vi "test Parse EST Clusters into EST IP.vi"(8 "error in (no error)":errorcluster, 11 "TestCase in":refnum<class "Bitfile Parsing Test Case.lvclass">) -> (0 "error out":errorcluster, 3 "TestCase out":refnum<class "Bitfile Parsing Test Case.lvclass">)   [LabVIEW 2015, in "Bitfile Parsing Test Case.lvclass"]
uses:
  Bitfile Parsing Test Case.lvclass
  <userlib>/_OpenG.lib/file/file.llb/Append Path to Root if Relative - Scalar__ogtk.vi
  <vilib>/addons/_JKI Toolkits/VI Tester/TestCase.llb/TestCase.lvclass
  System Explorer/Engine Simulation Toolkit System Explorer.lvlib
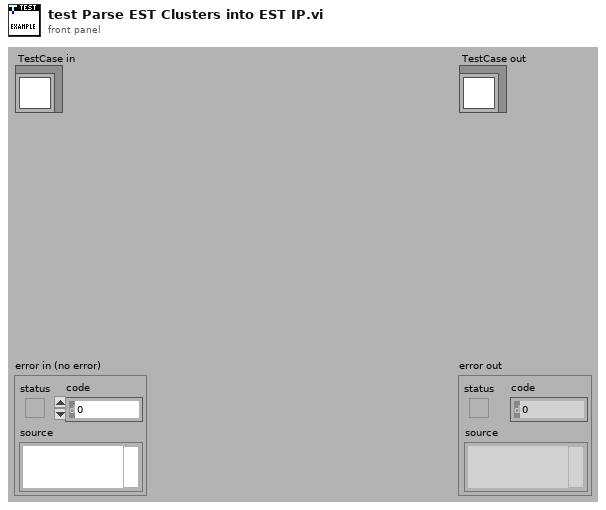
[diagram p1: front panel]
types:
  T1 = typedef "Engine Simulation Toolkit Shared.lvlib/Bitfile EST Version.ctl" = enum16{"1.0", "1.1", "1.2", "1.3"}
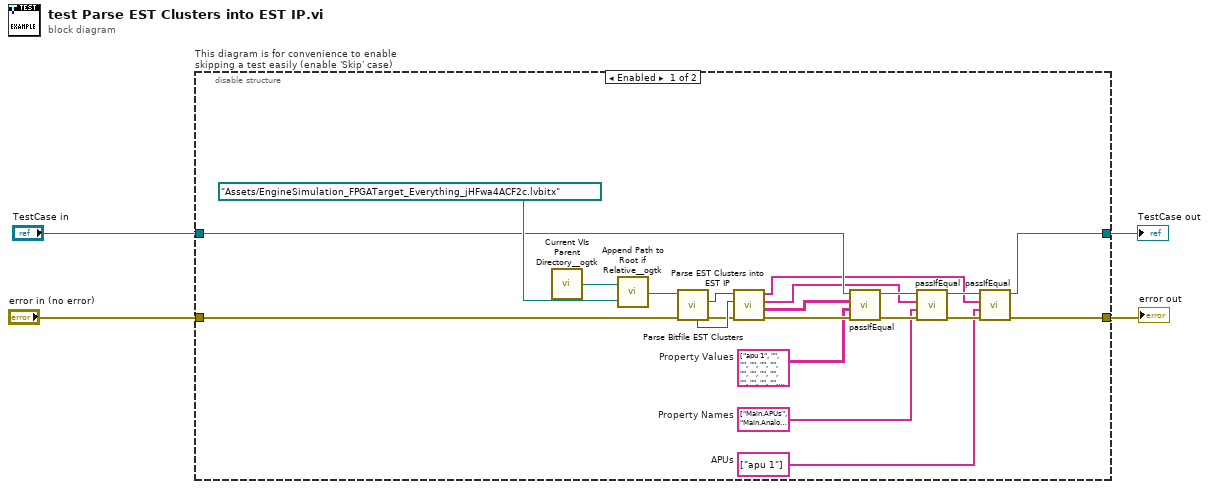
[diagram p0: block diagram]
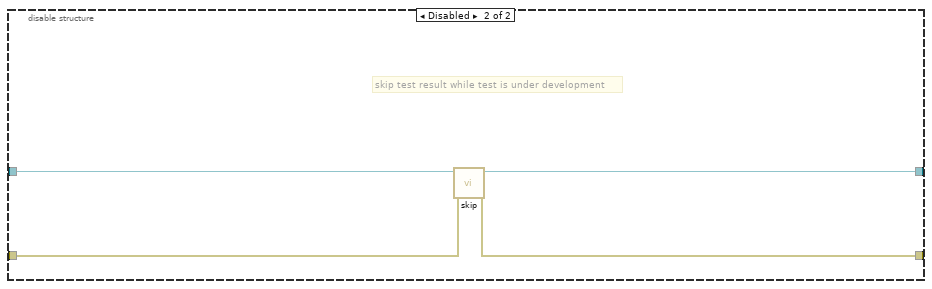
[diagram p2: hidden frame]
diagram:
  n1 = disable-structure "This diagram is for convenience to enable skipping a test easily (enable 'Skip' case)" shown="Enabled" {
    disable-tunnel: "TestCase in" -> [w17 w29]
    disable-tunnel: [w7 w27] -> w1
    disable-tunnel: [w9 w28] -> w3
    disable-tunnel: "error in (no error)" -> [w22 w26]
    frame Enabled {
      w16 = string[][] [["apu 1", "", "", "", "", "", "", "", "", "", "", "", "", "", "", "", "", "", "", "", "", "", "", "", "", "", "", "", "", ""], ["replay AO 0", "replay AO 1", "", "", "", "", "", "", "", "", "", "", "", "", "", "", "", "", "", "", "", "", "", "", "", "", "", "", "", ""], ["Pattern DIO 0", "Pattern DIO 1", "Pattern DIO 2", "Pattern DIO 3", "", "", "", "", "", "", "", "", "", "", "", "", "", "", "", "", "", "", "", "", "", "", "", "", "", ""], ["Event DIO 4.Event 1", "Event DIO 5.Event 1", "Event DIO 6.Event 1", "Event DIO 7.Event 1", "Event DIO 8.Event 1", "Event DIO 9.Event 1", "Multi Event DIO 10.Event 1", "Multi Event DIO 10.Event 2", "Multi Event DIO 10.Event 3", "Multi Event DIO 10.Event 4", "Multi Event DIO 11.Event 1", "Multi Event DIO 11.Event 2", "Multi Event DIO 11.Event 3", "Multi Event DIO 11.Event 4", "Multi Event DIO 12.Event 1", "Multi Event DIO 12.Event 2", "Multi Event DIO 12.Event 3", "Multi Event DIO 12.Event 4", "Multi Event DIO 13.Event 1", "Multi Event DIO 13.Event 2", "Multi Event DIO 13.Event 3", "Multi Event DIO 13.Event 4", "Multi Event DIO 14.Event 1", "Multi Event DIO 14.Event 2", "Multi Event DIO 14.Event 3", "Multi Event DIO 14.Event 4", "Multi Event DIO 15.Event 1", "Multi Event DIO 15.Event 2", "Multi Event DIO 15.Event 3", "Multi Event DIO 15.Event 4"], ["Event DIO 4", "Event DIO 5", "Event DIO 6", "Event DIO 7", "Event DIO 8", "Event DIO 9", "Multi Event DIO 10", "Multi Event DIO 11", "Multi Event DIO 12", "Multi Event DIO 13", "Multi Event DIO 14", "Multi Event DIO 15", "", "", "", "", "", "", "", "", "", "", "", "", "", "", "", "", "", ""], ["Knock AO 2.Cylinder 1", "Knock AO 2.Cylinder 2", "Knock AO 2.Cylinder 3", "Knock AO 2.Cylinder 4", "Knock AO 2.Cylinder 5", "Knock AO 2.Cylinder 6", "Knock AO 3.Cylinder 1", "Knock AO 3.Cylinder 2", "Knock AO 3.Cylinder 3", "Knock AO 3.Cylinder 4", "Knock AO 3.Cylinder 5", "Knock AO 3.Cylinder 6", "", "", "", "", "", "", "", "", "", "", "", "", "", "", "", "", "", ""], ["Knock AO 2", "Knock AO 3", "", "", "", "", "", "", "", "", "", "", "", "", "", "", "", "", "", "", "", "", "", "", "", "", "", "", "", ""], ["Dir Speed DIO0", "Dir Speed DIO1", "", "", "", "", "", "", "", "", "", "", "", "", "", "", "", "", "", "", "", "", "", "", "", "", "", "", "", ""]]  # Property Values
      w11 = string[] ["Main.APUs", "Main.Analog Replays", "Main.Digital PatGens", "Main.ETiming Caps", "Main.ETiming Meas", "Main.Knock Cylinder", "Main.Knock Sensor", "Main.DirSpeed Sensor"]  # Property Names
      w5 = string[] ["apu 1"]  # APUs
      n2 = call <userlib>:"Current VIs Parent Directory__ogtk.vi"() -> ("Parent Directory (+ Relative)"=w25:path)  [unwired: 5 in]
      n3 = call-poly <userlib>:"Append Path to Root if Relative__ogtk.vi"("Absolute or Relative Path"=path "Assets/EngineSimulation_FPGATarget_Everything_jHFwa4ACF2c.lvbitx" ("bitfile path"), "Root Path"=w25) -> ("Absolute or Appended Path"=w23:path)
      n4 = call "Parse Bitfile EST Clusters.vi"("error in (no error)"=w22, "bitfile path"=w23) -> ("error out"=w19:errorcluster, "EPS IP LUT"=w21:variant, "EST version enum"=w20:T1)  [unwired: 5 in, 2 out]
      n5 = call "Parse EST Clusters into EST IP.vi"("error in (no error)"=w19, "EST version enum"=w20, "EPS IP LUT"=w21) -> ("error out"=w18:errorcluster, "Property Values"=w15:string[][], "Property Names"=w12:string[], "APUs"=w6:string[])  [unwired: 5 in]
      n6 = call-dynamic "passIfEqual.vi"("error in (no error)"=w18, "y"=w16, "x"=w15, "TestCase in"=w17) -> ("error out"=w14:errorcluster, "TestCase out"=w13:refnum<class "Bitfile Parsing Test Case.lvclass">)  [unwired: 6 in]
      n7 = call-dynamic "passIfEqual.vi"("error in (no error)"=w14, "y"=w11, "x"=w12, "TestCase in"=w13) -> ("error out"=w10:errorcluster, "TestCase out"=w8:refnum<class "Bitfile Parsing Test Case.lvclass">)  [unwired: 6 in]
      n8 = call-dynamic "passIfEqual.vi"("error in (no error)"=w10, "y"=w5, "x"=w6, "TestCase in"=w8) -> ("error out"=w9:errorcluster, "TestCase out"=w7:refnum<class "Bitfile Parsing Test Case.lvclass">)  [unwired: 6 in]
    }
    frame Disabled {
      # "skip test result while test is under development"
      n9 = call <vilib>:"skip.vi"("error in (no error)"=w26, "TestCase in"=w29) -> ("error out"=w28:errorcluster, "TestCase out"=w27:refnum<class "Bitfile Parsing Test Case.lvclass">)  [unwired: 8 in]
    }
  }
  "error out" <- w3
  "TestCase out" <- w1
